vi "GUI_10TW_MAIN.vi"() -> ()   [LabVIEW 2013]
uses:
  shared programs/GUI_Template/GUI_master/tcp_new_data_event.ctl
  shared programs/GUI_Template/GUI_master/tcp new data cluster.ctl
panel:
  out "reading.var 6::13":dbl=1.515089 caption="Backing Pressure" min=-100000.0 max=100000.0 format="%#_4g"
  out "Backing Pressure":dbl
  in  "Last Motor Moved":string="JetZ"
  out "Latest Calibration":dbl=541835.0408322939
  in  "Latest Steps Moved":dbl=-25623.920916
  in  "Before Move":dbl=-0.419812
  out "Position.Axis 513::3":dbl caption="GodzZ" min=-999999.0 max=999999.0
  out "Position.Axis 443::3":dbl caption="PositionZ" min=-999999.0 max=999999.0
  out "Position.Axis 442::3":dbl caption="PositionY" min=-999999.0 max=999999.0
  out "reading.var 4::13":dbl=1.515089 caption="GodZ" min=-100000.0 max=100000.0 format="%#_4g"
  in  "Godz Cali":dbl
  in  "GodzZ":dbl=1.515089 format="%#_3g"
  in  "JetX":dbl=1.461297 format="%#.4f"
  in  "StepSize":dbl format="%#_4g"
  in  "JetZ":dbl=-0.46696 format="%.4f"
  in  "JetY":dbl=-1.85299 format="%#.4f"
  in  "Cali (stp/mm)":dbl=48444.0
  in  "RelativeSettings.Axis 3.StepSize::3":dbl caption="StepSizeZ" min=0.0 max=99999999.0
  in  "RelativeSettings.Axis 2.StepSize::3":dbl caption="StepSizeY" min=0.0 max=999999.0
  in  "RelativeSettings.Axis 1.StepSize::3":dbl caption="StepSizeX" min=0.0 max=999999.0
  out "Position.Axis 441::3":dbl caption="PositionX" min=-999999.0 max=999999.0
  in  "ActiveMotor":u16(ring) items=["Godzilla_M8_Steer (XH5/W)", "Godzilla_M6 (XHInt/W)", "Godzilla_M4 (XH3/XH4)", "Gas Jet", "Mode Imager"]
  in  "ActiveMotorName::3":string
  in  "GUIdevice 3":string="10TW_PicoPad1"
  in  "RelativeMove.Axis 3.CCW::3":bool caption="-Z"
  in  "RelativeMove.Axis 2.CCW::3":bool caption="-Y"
  in  "RelativeMove.Axis 2.CW::3":bool caption="+Y"
  in  "RelativeMove.Axis 1.CCW::3":bool caption="+X"
  in  "RelativeMove.Axis 1.CW::3":bool caption="-X"
  in  "RelativeMove.Axis 3.CW::3":bool caption="+Z"
  out "reading.var 3::13":dbl=-0.46696 caption="Gas Jet Z" min=-100000.0 max=100000.0 format="%#_4g"
  out "reading.var 2::13":dbl=-1.85299 caption="Gas Jet Y" min=-100000.0 max=100000.0 format="%#_3g"
  out "reading.var 1::13":dbl=1.461297 caption="Gas Jet X" min=-100000.0 max=100000.0 format="%#_4g"
  in  "Pressure.device 1::15":dbl=-0.5 caption="Gas Jet Press." min=0.0 max=250.0
  in  "Jet off":bool
  in  "GUIdevice 15":string="Alicat_10TW"
  in  "GUIdevice 13":string="10TW_DAQmultiplier"
  in  "stop":bool
  out "tcp data event":T1
  out "error IO 2":errorcluster
  # "General Pico Controls"
  # "Jet Controls"
  # "JetX"
  # "JetY"
  # "JetZ"
  # "Calibration (stp/mm)"
  # "GodZ"
  # "Calibration (stp/mm)"
  # "Step Size"
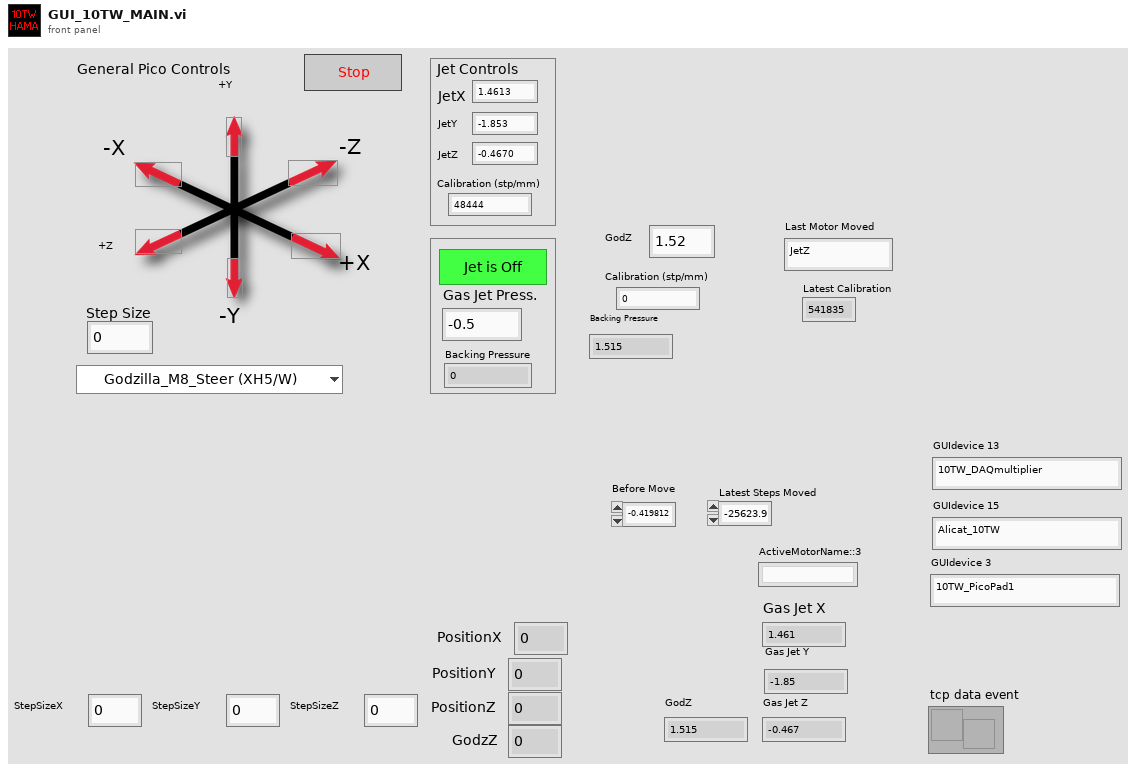
[diagram p1: front panel]
types:
  T1 = typedef "tcp_new_data_event.ctl" = refnum<user-event>
  T2 = typedef "tcp new data cluster.ctl" = cluster{"EventEnum":enum16{"new data", "connection status update"}, "Device name":string}
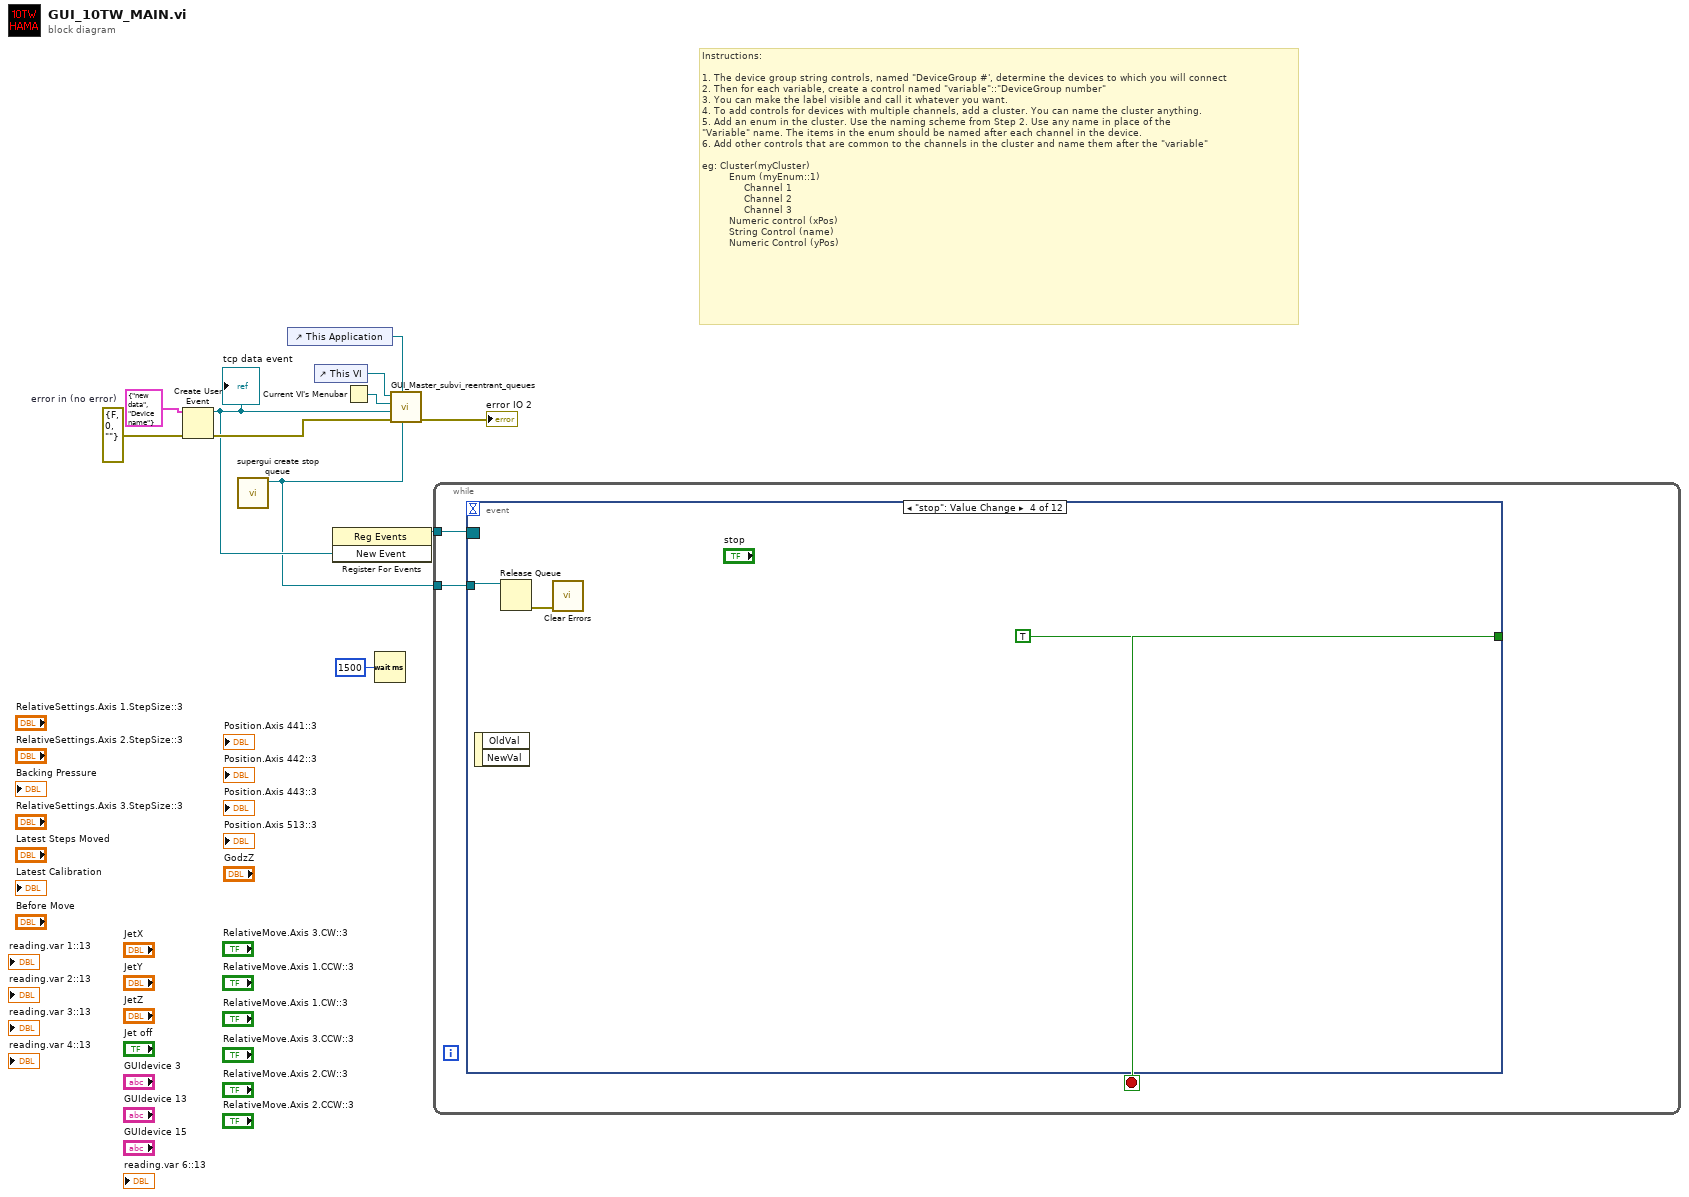
[diagram p0: block diagram]
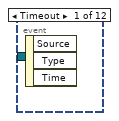
[diagram p2: hidden frame]
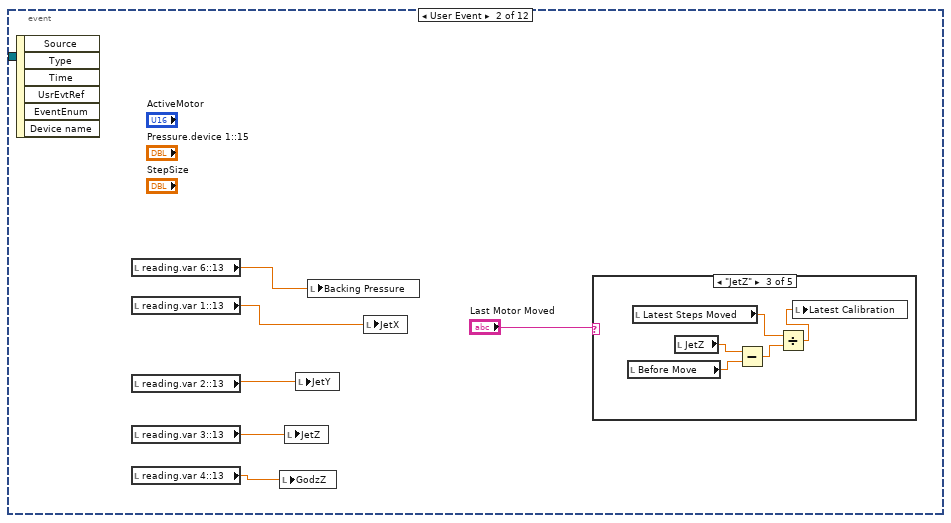
[diagram p3: hidden frame]
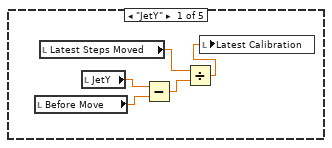
[diagram p4: hidden frame]
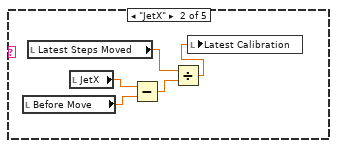
[diagram p5: hidden frame]
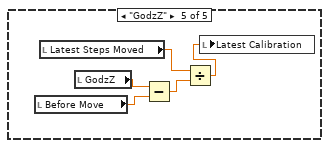
[diagram p7: hidden frame]
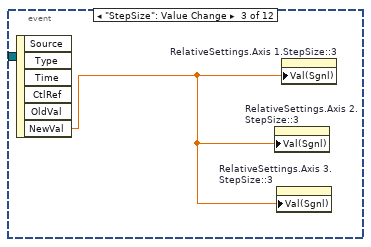
[diagram p8: hidden frame]
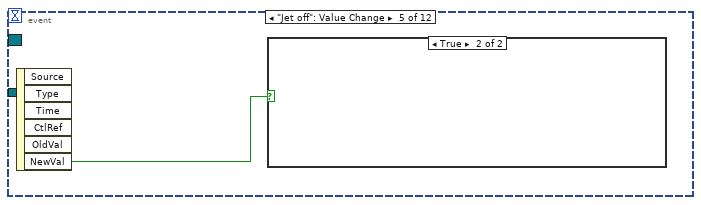
[diagram p9: hidden frame]
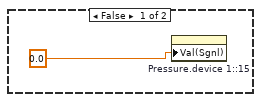
[diagram p10: hidden frame]
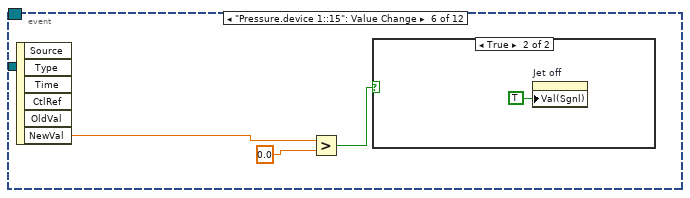
[diagram p11: hidden frame]
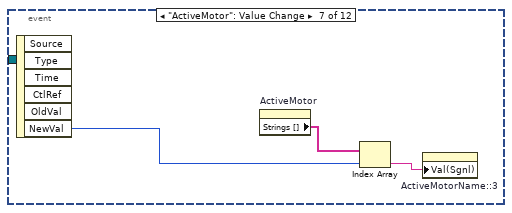
[diagram p13: hidden frame]
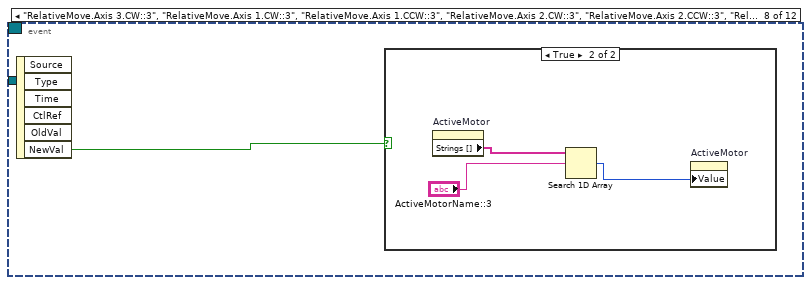
[diagram p14: hidden frame]
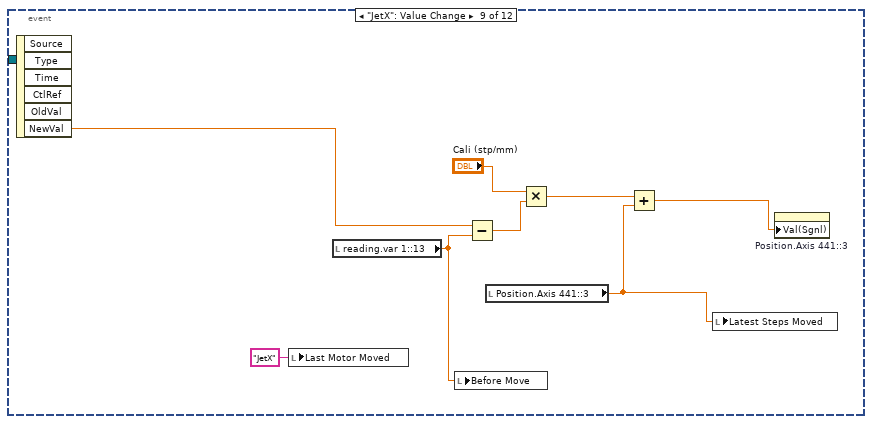
[diagram p16: hidden frame]
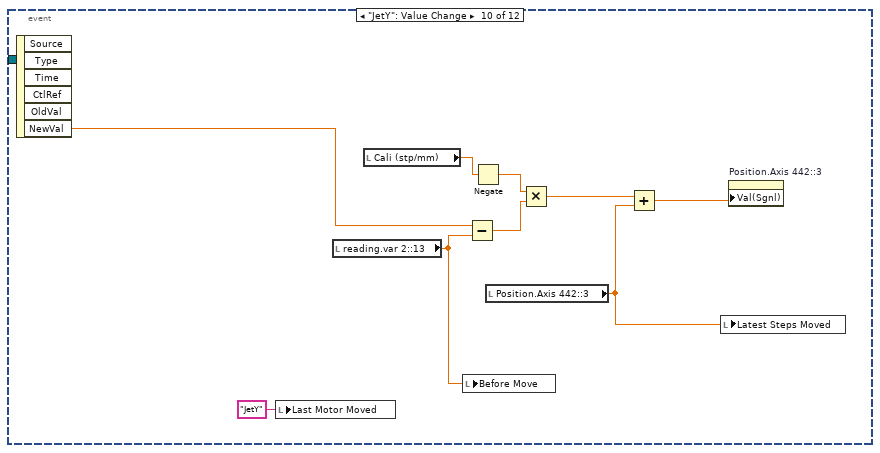
[diagram p17: hidden frame]
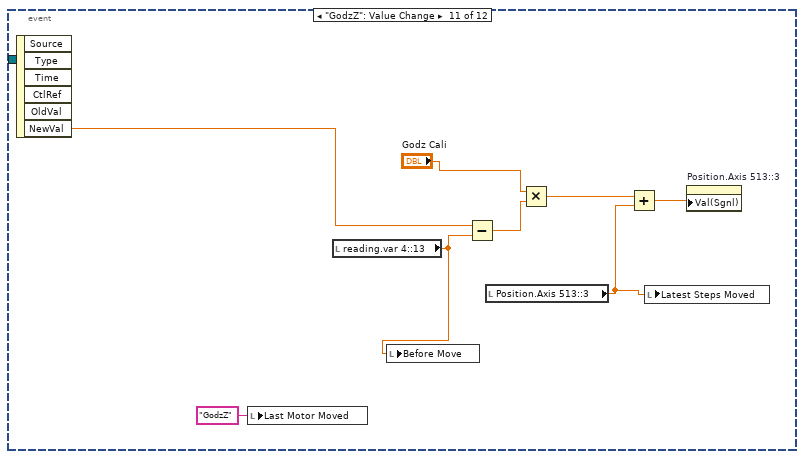
[diagram p18: hidden frame]
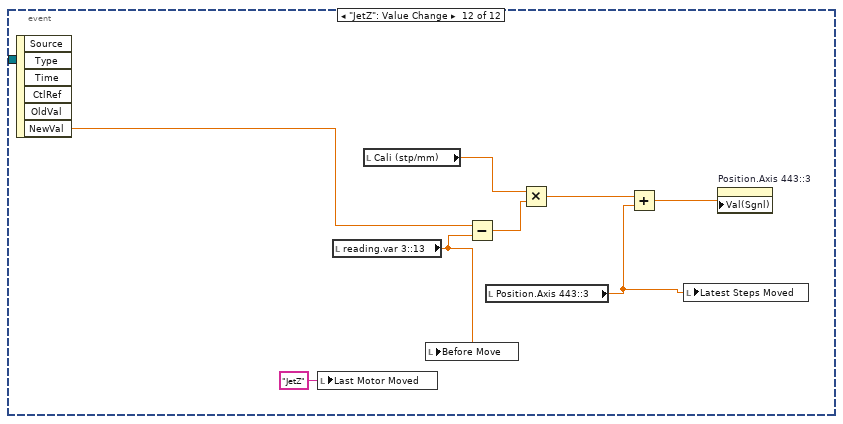
[diagram p19: hidden frame]
diagram:
  w5 = errorcluster {"status"=FALSE, "code"=0, "source"=""}  # error in (no error)
  # "Instructions:\n\n1. The device group string controls, named \"DeviceGroup #', determine the devices to which you will connect\n2. Then for each variable, create a control named \"variable\"::\"DeviceGroup number\"\n3. You can make the label visible and call it whatever you want.\n4. To add controls for devices with multiple channels, add a cluster. You can name the cluster anything.\n5. Add an enum in the cluster. Use the naming scheme from Step 2. Use any name in place of the \n\"Variable\" name. The items in the enum should be named after each channel in the device. \n6. Add other controls that are common to the channels in the cluster and name them after the \"variable\"\n\neg: Cluster(myCluster)\n         Enum (myEnum::1)\n              Channel 1 \n              Channel 2\n              Channel 3\n         Numeric control (xPos)\n         String Control (name)\n         Numeric Control (yPos)"
  n1 = Create User Event(user event datatype=T2 {"EventEnum"=enum."new data", "Device name"="Device name"} ("New Event"), error in=w5) -> (user event=w4:refnum<user-event>, error out=w7:errorcluster)
  "tcp data event" <- w4
  n2 = call "supergui create stop queue.vi"() -> ("STOP Queue out"=w1:refnum<queue>)  [unwired: 11 in]
  n3 = control-ref of="This Application"() -> (w6:refnum<vi>)
  n4 = control-ref of="This VI"() -> (w10:refnum<vi>)
  n5 = register-events(w4) -> (reference out=w3:refnum<event-registration>)  [unwired: 2 in, 1 out]
  n6 = Current VI's Menubar() -> (w9:refnum<k9>)
  n7 = Wait (ms)(milliseconds to wait=u32 1500) -> ()  [unwired: 1 out]
  n8 = call "GUI_Master_subvi_reentrant_queues.vi"("STOP Queue in"=w1, "This Application"=w6, "error in (no error)"=w7, "tcp data event"=w4, "Caller menu reference"=w9, "Caller VI ref"=w10) -> ("error out"=→"error IO 2":errorcluster)  [unwired: 5 in]
  n9 = while {
    tunnel: w3 -> [w14]
    tunnel: w1 -> [w12]
    stop <- w13 stop-if-true
    n10 = event shown="[3] \"stop\": Value Change" {
      selector: w14 -> [_ _ _ _ _ _ _ _ _ _ _ _]
      dyn-events: _ -> [_ _ _ _ _ _ _ _ _ _ _ _]
      timeout: _ -> [_ _ _ _ _ _ _ _ _ _ _ _]
      tunnel: [_ _ _ TRUE _ _ _ _ _ _ _ _] -> w13
      tunnel: w12 -> [_ _ _ w43 _ _ _ _ _ _ _ _]
      event Timeout {
        n11 = event-data() -> ()  [unwired: 1 in, 3 out]
      }
      event User Event {
        n12 = event-data() -> ()  [unwired: 1 in, 6 out]
        n13 = local read "reading.var 6::13"() -> (w15:dbl)
        n14 = local read "reading.var 1::13"() -> (w20:dbl)
        n15 = local read "reading.var 2::13"() -> (w19:dbl)
        n16 = local read "reading.var 3::13"() -> (w18:dbl)
        n17 = local read "reading.var 4::13"() -> (w17:dbl)
        n18 = local write "GodzZ"(w17) -> ()
        n19 = local write "JetZ"(w18) -> ()
        n20 = local write "JetY"(w19) -> ()
        n21 = local write "Backing Pressure"(w15) -> ()
        n22 = local write "JetX"(w20) -> ()
        n23 = case shown="\"JetZ\"" "Last Motor Moved" {
          frame "JetY" {
            n24 = local read "Before Move"() -> (w24:dbl)
            n25 = local read "Latest Steps Moved"() -> (w23:dbl)
            n26 = local read "JetY"() -> (w25:dbl)
            n27 = Subtract(x=w25, y=w24) -> (x-y=w22:dbl)
            n28 = Divide(x=w23, y=w22) -> (x/y=w21:dbl)
            n29 = local write "Latest Calibration"(w21) -> ()
          }
          frame "JetX" {
            n30 = local read "Before Move"() -> (w29:dbl)
            n31 = local read "Latest Steps Moved"() -> (w28:dbl)
            n32 = local read "JetX"() -> (w30:dbl)
            n33 = Subtract(x=w30, y=w29) -> (x-y=w27:dbl)
            n34 = Divide(x=w28, y=w27) -> (x/y=w26:dbl)
            n35 = local write "Latest Calibration"(w26) -> ()
          }
          frame "JetZ" {
            n36 = local read "Before Move"() -> (w34:dbl)
            n37 = local read "Latest Steps Moved"() -> (w33:dbl)
            n38 = local read "JetZ"() -> (w35:dbl)
            n39 = Subtract(x=w35, y=w34) -> (x-y=w32:dbl)
            n40 = Divide(x=w33, y=w32) -> (x/y=w31:dbl)
            n41 = local write "Latest Calibration"(w31) -> ()
          }
          frame "", Default {
          }
          frame "GodzZ" {
            n42 = local read "Before Move"() -> (w39:dbl)
            n43 = local read "Latest Steps Moved"() -> (w38:dbl)
            n44 = local read "GodzZ"() -> (w40:dbl)
            n45 = Subtract(x=w40, y=w39) -> (x-y=w37:dbl)
            n46 = Divide(x=w38, y=w37) -> (x/y=w36:dbl)
            n47 = local write "Latest Calibration"(w36) -> ()
          }
        }
      }
      event "StepSize": Value Change {
        n48 = event-data() -> ("NewVal"=w41:dbl)  [unwired: 1 in, 5 out]
        n49 = property on="RelativeSettings.Axis 2.StepSize::3" class="DigNum (strict)"("Val(Sgnl)"=w41) -> ()  [unwired: 2 in, 2 out]
        n50 = property on="RelativeSettings.Axis 3.StepSize::3" class="DigNum (strict)"("Val(Sgnl)"=w41) -> ()  [unwired: 2 in, 2 out]
        n51 = property on="RelativeSettings.Axis 1.StepSize::3" class="DigNum (strict)"("Val(Sgnl)"=w41) -> ()  [unwired: 2 in, 2 out]
      }
      event "stop": Value Change {
        n52 = event-data() -> ()  [unwired: 1 in, 2 out]
        n53 = Release Queue(queue=w43) -> (error out=w42:errorcluster)  [unwired: 2 in, 2 out]
        n54 = call <vilib>:"Clear Errors.vi"("error in (no error)"=w42) -> ()  [unwired: 6 in, 1 out]
      }
      event "Jet off": Value Change {
        n55 = event-data() -> ("NewVal"=w45:bool)  [unwired: 1 in, 5 out]
        n56 = case shown="True" w45 {
          frame False {
            n57 = property on="Pressure.device 1::15" class="DigNum (strict)"("Val(Sgnl)"=0.0 ("Pressure.device 1::15")) -> ()  [unwired: 2 in, 2 out]
          }
          frame True {
          }
        }
      }
      event "Pressure.device 1::15": Value Change {
        n58 = event-data() -> ("NewVal"=w48:dbl)  [unwired: 1 in, 5 out]
        n59 = Greater?(x=w48, y=0.0) -> (0:w47:bool)
        n60 = case shown="True" w47 {
          frame False {
          }
          frame True {
            n61 = property on="Jet off" class="Bool (strict)"("Val(Sgnl)"=TRUE ("Value (Signaling)")) -> ()  [unwired: 2 in, 2 out]
          }
        }
      }
      event "ActiveMotor": Value Change {
        n62 = event-data() -> ("NewVal"=w53:u16)  [unwired: 1 in, 5 out]
        n63 = property on="ActiveMotor" class="Ring (strict)"() -> ("Strings []"=w52:string[])  [unwired: 2 in, 2 out]
        n64 = Index Array(array=w52, index=w53) -> (element=w51:string)
        n65 = property on="ActiveMotorName::3" class="Str"("Val(Sgnl)"=w51) -> ()  [unwired: 2 in, 2 out]
      }
      event "RelativeMove.Axis 3.CW::3", "RelativeMove.Axis 1.CW::3", "RelativeMove.Axis 1.CCW::3", "RelativeMove.Axis 2.CW::3", "RelativeMove.Axis 2.CCW::3", "RelativeMove.Axis 3.CCW::3": Value Change {
        n66 = event-data() -> ("NewVal"=w54:bool)  [unwired: 1 in, 5 out]
        n67 = case shown="True" w54 {
          frame False {
          }
          frame True {
            n68 = property on="ActiveMotor" class="Ring (strict)"() -> ("Strings []"=w57:string[])  [unwired: 2 in, 2 out]
            n69 = Search 1D Array(1D array=w57, element="ActiveMotorName::3") -> (index of element=w55:i32)  [unwired: 1 in]
            n70 = property on="ActiveMotor" class="Ring (strict)"("Value"=w55) -> ()  [unwired: 2 in, 2 out]
          }
        }
      }
      event "JetX": Value Change {
        n71 = event-data() -> ("NewVal"=w65:dbl)  [unwired: 1 in, 5 out]
        n72 = local write "Last Motor Moved"("JetX" ("Last Motor Moved")) -> ()
        n73 = local read "reading.var 1::13"() -> (w60:dbl)
        n74 = local write "Before Move"(w60) -> ()
        n75 = Subtract(x=w65, y=w60) -> (x-y=w63:dbl)
        n76 = local read "Position.Axis 441::3"() -> (w59:dbl)
        n77 = Multiply(x="Cali (stp/mm)", y=w63) -> (x*y=w64:dbl)
        n78 = Add(x=w64, y=w59) -> (x+y=w61:dbl)
        n79 = local write "Latest Steps Moved"(w59) -> ()
        n80 = property on="Position.Axis 441::3" class="DigNum (strict)"("Val(Sgnl)"=w61) -> ()  [unwired: 2 in, 2 out]
      }
      event "JetY": Value Change {
        n81 = event-data() -> ("NewVal"=w74:dbl)  [unwired: 1 in, 5 out]
        n82 = local write "Last Motor Moved"("JetY" ("Last Motor Moved")) -> ()
        n83 = local read "reading.var 2::13"() -> (w68:dbl)
        n84 = local read "Cali (stp/mm)"() -> (w71:dbl)
        n85 = local write "Before Move"(w68) -> ()
        n86 = Subtract(x=w74, y=w68) -> (x-y=w72:dbl)
        n87 = Negate(x=w71) -> (-x=w70:dbl)
        n88 = local read "Position.Axis 442::3"() -> (w67:dbl)
        n89 = Multiply(x=w70, y=w72) -> (x*y=w73:dbl)
        n90 = Add(x=w73, y=w67) -> (x+y=w69:dbl)
        n91 = local write "Latest Steps Moved"(w67) -> ()
        n92 = property on="Position.Axis 442::3" class="DigNum (strict)"("Val(Sgnl)"=w69) -> ()  [unwired: 2 in, 2 out]
      }
      event "GodzZ": Value Change {
        n93 = event-data() -> ("NewVal"=w82:dbl)  [unwired: 1 in, 5 out]
        n94 = local write "Last Motor Moved"("GodzZ" ("Last Motor Moved")) -> ()
        n95 = local read "reading.var 4::13"() -> (w77:dbl)
        n96 = local write "Before Move"(w77) -> ()
        n97 = Subtract(x=w82, y=w77) -> (x-y=w80:dbl)
        n98 = local read "Position.Axis 513::3"() -> (w76:dbl)
        n99 = Multiply(x="Godz Cali", y=w80) -> (x*y=w81:dbl)
        n100 = Add(x=w81, y=w76) -> (x+y=w78:dbl)
        n101 = local write "Latest Steps Moved"(w76) -> ()
        n102 = property on="Position.Axis 513::3" class="DigNum (strict)"("Val(Sgnl)"=w78) -> ()  [unwired: 2 in, 2 out]
      }
      event "JetZ": Value Change {
        n103 = event-data() -> ("NewVal"=w86:dbl)  [unwired: 1 in, 5 out]
        n104 = local write "Last Motor Moved"("JetZ" ("Last Motor Moved")) -> ()
        n105 = local read "reading.var 3::13"() -> (w84:dbl)
        n106 = local read "Cali (stp/mm)"() -> (w88:dbl)
        n107 = local write "Before Move"(w84) -> ()
        n108 = Subtract(x=w86, y=w84) -> (x-y=w89:dbl)
        n109 = local read "Position.Axis 443::3"() -> (w85:dbl)
        n110 = Multiply(x=w88, y=w89) -> (x*y=w90:dbl)
        n111 = Add(x=w90, y=w85) -> (x+y=w87:dbl)
        n112 = local write "Latest Steps Moved"(w85) -> ()
        n113 = property on="Position.Axis 443::3" class="DigNum (strict)"("Val(Sgnl)"=w87) -> ()  [unwired: 2 in, 2 out]
      }
    }
  }
